vi "Search Array of Strings.vi"(10 "search string":string, 11 "Search array":string[](array[string])) -> (2 "found elements":string[](array[string]), 3 "indices":i32[](array[numeric]))   [LabVIEW 2026, in "TALOS.lvlib"]
doc: "Apparently this is the most efficient way of searching an array of strings (https://lavag.org/topic/15969-fastest-search-array-of-string/)."
uses:
  TALOS.lvlib
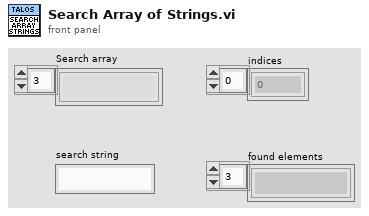
[diagram p1: front panel]
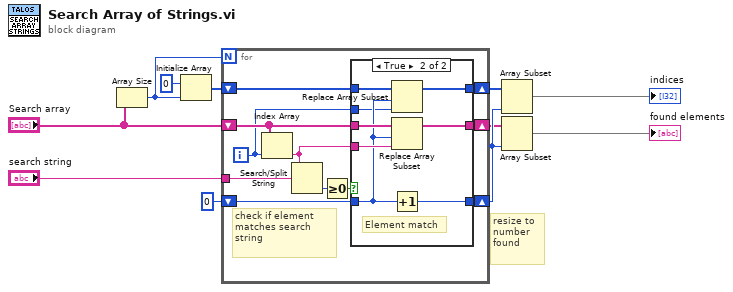
[diagram p0: block diagram]
diagram:
  # "resize to number found"
  n1 = Array Size(array="Search array") -> (size(s)=w6:i32)
  n2 = Initialize Array(0, w6) -> (w4:i32[])
  n3 = for {
    N: w6 -> [_]
    shift-right: [w18] -> w8
    shift-left: "Search array" -> [w19]
    shift-right: [w15] -> w9
    shift-left: 0 -> [w20]
    tunnel: "search string" -> [w21]
    shift-right: [w13] -> w7
    shift-left: w4 -> [w14]
    i -> [w12]
    # "check if element matches search string"
    n4 = Index Array(array=w19, index=w12) -> (element=w22:string)
    n5 = Search/Split String(string=w22, search string/char (-)=w21) -> (offset of match=w17:i32)  [unwired: 1 in, 2 out]
    n6 = Greater Or Equal To 0?(x=w17) -> (x >= 0?=w16:bool)
    n7 = case shown="True" w16 {
      tunnel: w22 -> [_ w33]
      tunnel: w20 -> [w24 w27]
      tunnel: w19 -> [w25 w32]
      tunnel: [w25 w31] -> w18
      tunnel: [w24 w30] -> w15
      tunnel: w14 -> [w23 w29]
      tunnel: [w23 w28] -> w13
      tunnel: w12 -> [_ w26]
      frame False {
        # "no match"
      }
      frame True {
        # "Element match"
        n8 = Replace Array Subset(array=w29, new element=w26, index=w27) -> (w28:i32[])
        n9 = Replace Array Subset(array=w32, new element=w33, index=w27) -> (w31:string[])
        n10 = Increment(x=w27) -> (x+1=w30:i32)
      }
    }
  }
  n11 = Array Subset(array=w7, length=w9) -> (→"indices":i32[])  [unwired: 1 in]
  n12 = Array Subset(array=w8, length=w9) -> (→"found elements":string[])  [unwired: 1 in]
